vi "Main.vi"   [LabVIEW 2021]
uses:
  Dev Actor/Dev Actor/Dev Actor.lvclass
  C:/Program Files/National Instruments/LabVIEW 2021/vi.lib/jettl/jettl/jettl/Actor/Actor.lvclass
  <vilib>/jettl/jettl/jettl/Self Actor/Self Actor.lvclass
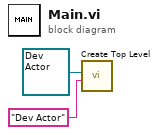
[diagram p0: block diagram]
diagram:
  n1 = call <vilib>:"Create Top Level.vi"("Alias"="Dev Actor", "Actor"=refnum<class "Dev Actor.lvclass"> refnum ("Process.lvlib:Process.lvclass")) -> ()  [unwired: 10 in]
